vi "Carbon - Send Command.vi"(8 "error in (no error)":errorcluster, 10 "Password":string, 11 "Carbon Command":string=" qstat") -> (0 "error out":errorcluster, 2 "Error String":string, 3 "Output String":string)   [LabVIEW 2010]
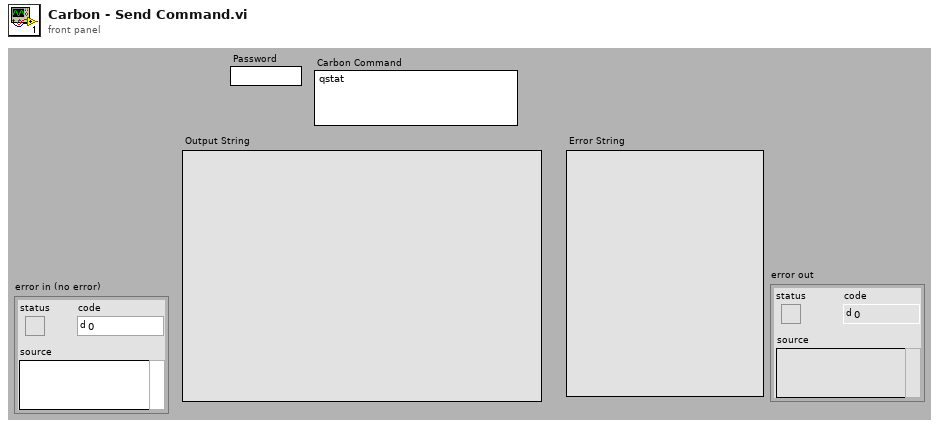
[diagram p1: front panel]
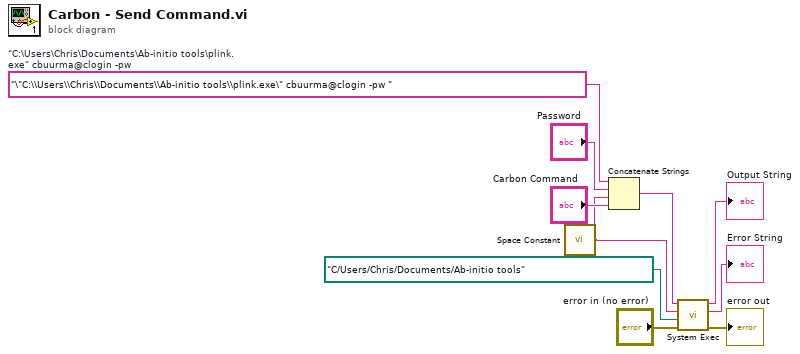
[diagram p0: block diagram]
diagram:
  w9 = "\"C:\\Users\\Chris\\Documents\\Ab-initio tools\\plink.exe\" cbuurma@clogin -pw "  # "C:\Users\Chris\Documents\Ab-initio tools\plink.exe" cbuurma@clogin -pw
  n1 = call <vilib>:"Space Constant.vi"() -> ("String"=w3:string)
  n2 = Concatenate Strings(w9, "Password", w3, "Carbon Command") -> (w7:string)
  n3 = call <vilib>:"System Exec.vi"("error in (no error)"="error in (no error)", "working directory"=path "C:/Users/Chris/Documents/Ab-initio tools", "standard input"=w3, "command line"=w7) -> ("error out"=→"error out":errorcluster, "standard error"=→"Error String":string, "standard output"=→"Output String":string)  [unwired: 4 in, 1 out]
